vi "SwrvLinAlg Wheel Angles.vi"(8 "Rotate In":dbl, 10 "x,y movement vector":dbl[](array[numeric]), 11 "Theta":dbl) -> (0 "BR Final":dbl[](array[numeric]), 1 "BL Final":dbl[](array[numeric]), 2 "FR Final":dbl[](array[numeric]), 3 "FL Final":dbl[](array[numeric]))   [LabVIEW 2017]
uses:
  <vilib>/Analysis/baseanly.llb/A x B.vi
  <vilib>/Analysis/baseanly.llb/A x Vector.vi
panel:
  out "BR Rotate":dbl[](array[numeric])
  out "BL Rotate":dbl[](array[numeric])
  out "FR Rotate":dbl[](array[numeric])
  out "FL Rotate":dbl[](array[numeric])
  out "Solution Vector":dbl[](array[numeric]) format="%.2f"
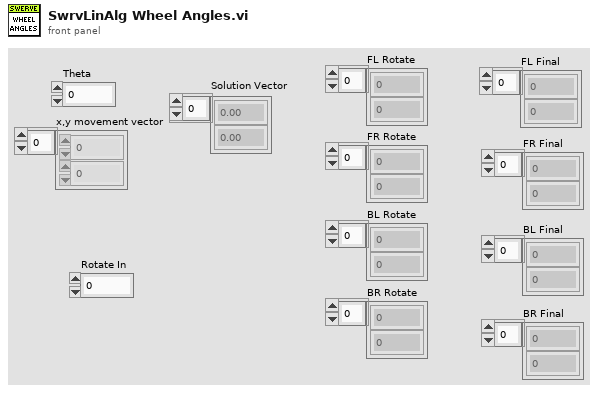
[diagram p1: front panel]
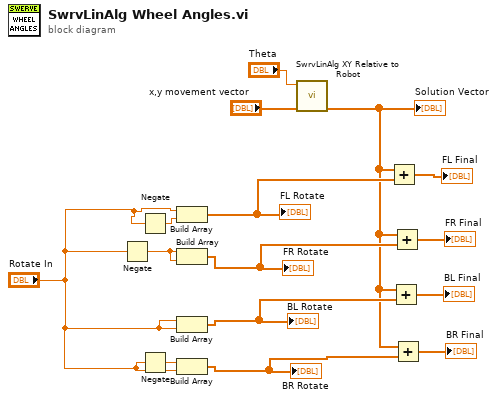
[diagram p0: block diagram]
diagram:
  n1 = Negate(x="Rotate In") -> (-x=w3:dbl)
  n2 = Negate(x="Rotate In") -> (-x=w2:dbl)
  n3 = Negate(x="Rotate In") -> (-x=w4:dbl)
  n4 = Build Array("Rotate In", w2) -> (w15:dbl[])
  "FL Rotate" <- w15
  n5 = Build Array(w3, w3) -> (w10:dbl[])
  "FR Rotate" <- w10
  n6 = Build Array("Rotate In", "Rotate In") -> (w9:dbl[])
  "BL Rotate" <- w9
  n7 = Build Array(w4, "Rotate In") -> (w8:dbl[])
  "BR Rotate" <- w8
  n8 = call "SwrvLinAlg XY Relative to Robot.vi"("x,y movement vector"="x,y movement vector", "Theta"="Theta") -> ("A x Vector"=w7:dbl[])  [unwired: 8 in, 1 out]
  "Solution Vector" <- w7
  n9 = Add(x=w7, y=w15) -> (x+y=→"FL Final":dbl[])
  n10 = Add(x=w7, y=w9) -> (x+y=→"BL Final":dbl[])
  n11 = Add(x=w7, y=w10) -> (x+y=→"FR Final":dbl[])
  n12 = Add(x=w7, y=w8) -> (x+y=→"BR Final":dbl[])
